vi "String to Enum Example.vi"() -> ()   [LabVIEW 2017]
uses:
  <userlib>/_NEVSTOP/Communicable State Machine(CSM)/Communicable State Machine.lvlib
  API-String-Arugments-Support/API String Arguments Support.lvlib
panel:
  out "Array 4":T1(array[ring])
  out "Array 3":T1(array[ring])
  out "Array 2":T2(array[ring])
  out "data 7":T3(array[ring])
  out "Array":T2(array[ring])
  out "data 6":T3(array[ring])
  out "data 4":T4(ring)
  out "data 3":T5(ring)
  out "data 2":T5(ring)
  out "data":T4(ring)
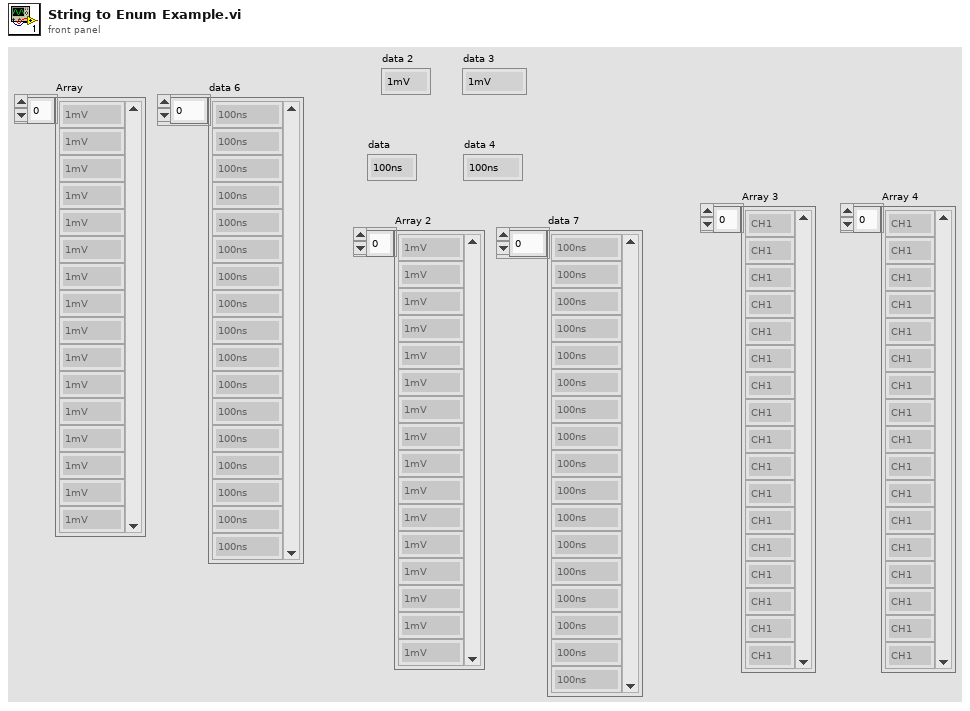
[diagram p1: front panel]
types:
  T1 = enum16{"CH1", "CH2", "CH3", "CH4", "CH5", "CH6", "CH7", "CH8", "CH9", "CH10", "CH11", "CH12", "CH13", "CH14", "CH15", "CH16"}[]
  T2 = enum16{"1mV", "2mV", "5mV", "10mV", "20mV", "50mV", "100mV", "200mV", "500mV", "1V", "2V", "5V", "10V", "20V", "50V", "100V", "200V", "500V", "1kV", "2kV", "5kV", "10kV", "20kV"}[]
  T3 = enum16{"100ns", "200ns", "500ns", "1us", "2us", "5us", "10us", "20us", "50us", "100us", "200us", "500us", "1ms", "2ms", "5ms", "10ms", "20ms", "50ms", "100ms", "200ms", "500ms", "1s", "2s", "3s", "4s", "5s", "6s", "8s", "10s", "20s", "30s", "1min", "2min", "3min", "4min", "5min", "6min", "7min", "8min", "9min", "10min", "12min", "15min", "30min", "1hour", "2hour", "3hour", "4hour", "5hour", "6hour", "7hour", "8hour", "9hour", "10hour", "12hour", "1day", "2day", "3day"}[]
  T4 = enum16{"100ns", "200ns", "500ns", "1us", "2us", "5us", "10us", "20us", "50us", "100us", "200us", "500us", "1ms", "2ms", "5ms", "10ms", "20ms", "50ms", "100ms", "200ms", "500ms", "1s", "2s", "3s", "4s", "5s", "6s", "8s", "10s", "20s", "30s", "1min", "2min", "3min", "4min", "5min", "6min", "7min", "8min", "9min", "10min", "12min", "15min", "30min", "1hour", "2hour", "3hour", "4hour", "5hour", "6hour", "7hour", "8hour", "9hour", "10hour", "12hour", "1day", "2day", "3day"}
  T5 = enum16{"1mV", "2mV", "5mV", "10mV", "20mV", "50mV", "100mV", "200mV", "500mV", "1V", "2V", "5V", "10V", "20V", "50V", "100V", "200V", "500V", "1kV", "2kV", "5kV", "10kV", "20kV"}
  T6 = enum16{"CH1", "CH2", "CH3", "CH4", "CH5", "CH6", "CH7", "CH8", "CH9", "CH10", "CH11", "CH12", "CH13", "CH14", "CH15", "CH16"}
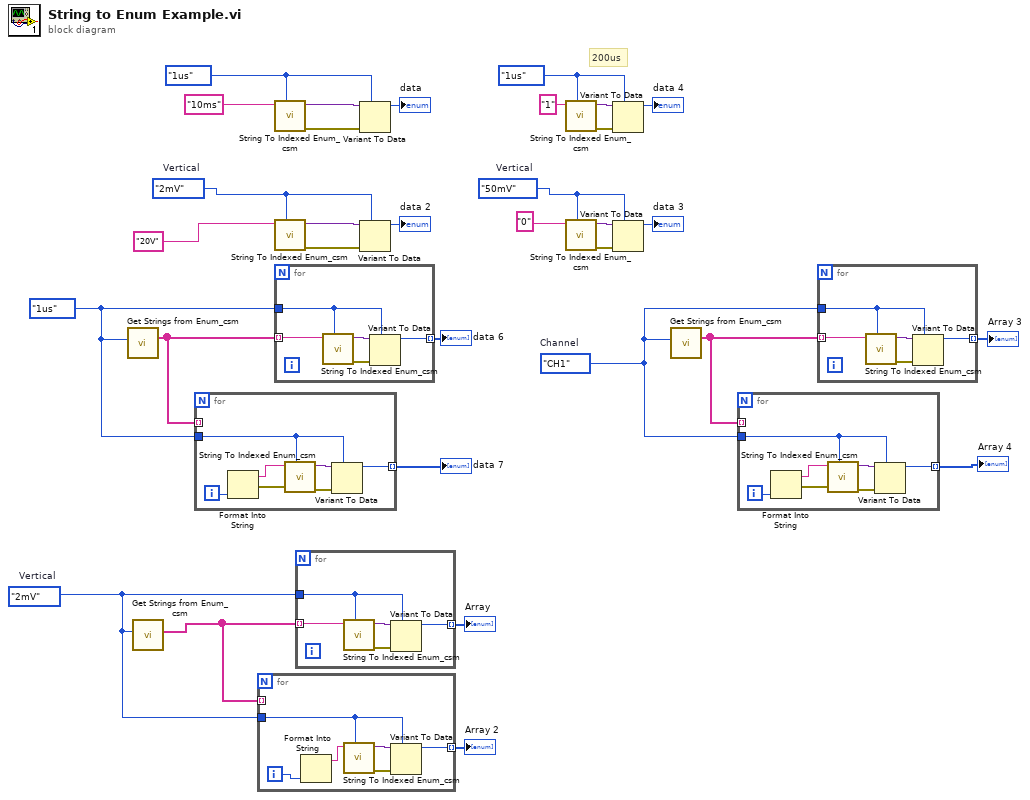
[diagram p0: block diagram]
diagram:
  w3 = T6."CH1"  # Channel
  w8 = T4."1us" ("Time/Division (12: 1ms)")
  w5 = T5."2mV"  # Vertical
  w15 = T4."1us" ("Time/Division (12: 1ms)")
  w21 = T5."50mV"  # Vertical
  w30 = T4."1us" ("Time/Division (12: 1ms)")
  w24 = T5."2mV"  # Vertical
  # "200us"
  n1 = call <userlib>:"Get Strings from Enum_csm.vi"("Enum"=w8) -> ("Enum Strings"=w7:string[])  [unwired: 7 in, 3 out]
  n2 = call <userlib>:"Get Strings from Enum_csm.vi"("Enum"=w5) -> ("Enum Strings"=w6:string[])  [unwired: 7 in, 3 out]
  n3 = for {
    tunnel: w8 -> [w37]
    tunnel: [w36] -> w9 mode=indexing
    tunnel: w7 -> [_] mode=indexing
    i -> [w34]
    n4 = Format Into String(w34) -> (resulting string=w33:string, error out=w35:errorcluster)  [unwired: 3 in]
    n5 = call "String To Indexed Enum_csm.vi"("Variant"=w37, "error in (no error)"=w35, "String"=w33) -> ("error out"=w38:errorcluster, "Enum"=w39:variant)  [unwired: 7 in]
    n6 = Variant To Data(error in=w38, type=w37, Variant=w39) -> (data=w36:T4)  [unwired: 1 out]
  }
  "data 7" <- w9
  n7 = for {
    tunnel: w5 -> [w43]
    tunnel: [w42] -> w10 mode=indexing
    tunnel: w6 -> [_] mode=indexing
    i -> [w41]
    n8 = Format Into String(w41) -> (resulting string=w40:string)  [unwired: 3 in, 1 out]
    n9 = call "String To Indexed Enum_csm.vi"("Variant"=w43, "String"=w40) -> ("error out"=w44:errorcluster, "Enum"=w45:variant)  [unwired: 8 in]
    n10 = Variant To Data(error in=w44, type=w43, Variant=w45) -> (data=w42:T5)  [unwired: 1 out]
  }
  "Array 2" <- w10
  n11 = call "String To Indexed Enum_csm.vi"("Variant"=w30, "String"="10ms") -> ("error out"=w32:errorcluster, "Enum"=w31:variant)  [unwired: 8 in]
  n12 = call "String To Indexed Enum_csm.vi"("Variant"=w24, "String"="20V") -> ("error out"=w25:errorcluster, "Enum"=w26:variant)  [unwired: 8 in]
  n13 = for {
    tunnel: w8 -> [w48]
    tunnel: w7 -> [w47] mode=indexing
    tunnel: [w46] -> w12 mode=indexing
    n14 = call "String To Indexed Enum_csm.vi"("Variant"=w48, "String"=w47) -> ("error out"=w49:errorcluster, "Enum"=w50:variant)  [unwired: 8 in]
    n15 = Variant To Data(error in=w49, type=w48, Variant=w50) -> (data=w46:T4)  [unwired: 1 out]
  }
  "data 6" <- w12
  n16 = for {
    tunnel: w5 -> [w53]
    tunnel: w6 -> [w52] mode=indexing
    tunnel: [w51] -> w11 mode=indexing
    n17 = call "String To Indexed Enum_csm.vi"("Variant"=w53, "String"=w52) -> ("error out"=w54:errorcluster, "Enum"=w55:variant)  [unwired: 8 in]
    n18 = Variant To Data(error in=w54, type=w53, Variant=w55) -> (data=w51:T5)  [unwired: 1 out]
  }
  "Array" <- w11
  n19 = Variant To Data(error in=w32, type=w30, Variant=w31) -> (data=→"data":T4)  [unwired: 1 out]
  n20 = Variant To Data(error in=w25, type=w24, Variant=w26) -> (data=→"data 2":T5)  [unwired: 1 out]
  n21 = call "String To Indexed Enum_csm.vi"("Variant"=w15, "String"="1") -> ("error out"=w13:errorcluster, "Enum"=w14:variant)  [unwired: 8 in]
  n22 = call "String To Indexed Enum_csm.vi"("Variant"=w21, "String"="0") -> ("error out"=w20:errorcluster, "Enum"=w19:variant)  [unwired: 8 in]
  n23 = Variant To Data(error in=w13, type=w15, Variant=w14) -> (data=→"data 4":T4)  [unwired: 1 out]
  n24 = Variant To Data(error in=w20, type=w21, Variant=w19) -> (data=→"data 3":T5)  [unwired: 1 out]
  n25 = call <userlib>:"Get Strings from Enum_csm.vi"("Enum"=w3) -> ("Enum Strings"=w4:string[])  [unwired: 7 in, 3 out]
  n26 = for {
    tunnel: w3 -> [w60]
    tunnel: [w59] -> w1 mode=indexing
    tunnel: w4 -> [_] mode=indexing
    i -> [w57]
    n27 = Format Into String(w57) -> (resulting string=w56:string, error out=w58:errorcluster)  [unwired: 3 in]
    n28 = call "String To Indexed Enum_csm.vi"("Variant"=w60, "error in (no error)"=w58, "String"=w56) -> ("error out"=w61:errorcluster, "Enum"=w62:variant)  [unwired: 7 in]
    n29 = Variant To Data(error in=w61, type=w60, Variant=w62) -> (data=w59:T6)  [unwired: 1 out]
  }
  "Array 4" <- w1
  n30 = for {
    tunnel: w3 -> [w65]
    tunnel: w4 -> [w64] mode=indexing
    tunnel: [w63] -> w2 mode=indexing
    n31 = call "String To Indexed Enum_csm.vi"("Variant"=w65, "String"=w64) -> ("error out"=w66:errorcluster, "Enum"=w67:variant)  [unwired: 8 in]
    n32 = Variant To Data(error in=w66, type=w65, Variant=w67) -> (data=w63:T6)  [unwired: 1 out]
  }
  "Array 3" <- w2
